vi "GlobalFavoritesList.vi"() -> ()   [LabVIEW 2013]
panel:
  in  "Favorite param number":dbl[](array[numeric])
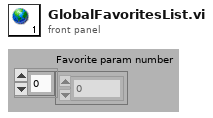
[diagram p1: front panel]
diagram:
